vi "Set SPAN Component Lin.vi"(10 "LIN":T1, 11 "Lin Offset Cluster":T3) -> ()   [LabVIEW 2020, in "Linearisierung v2.lvlib" / "SpanEinstellungen.lvlib"]
uses:
  SpanEinstellungen.lvlib
  Auswahl Polynom Ordnung.ctl
  Linearisierung v2.lvlib
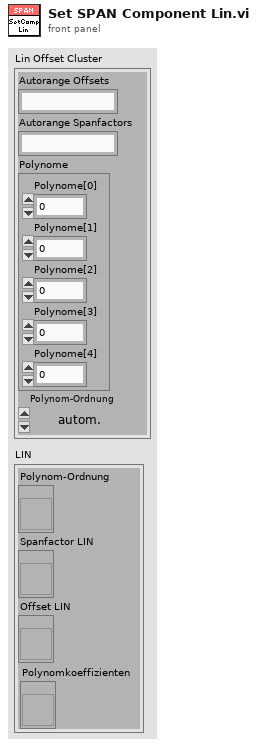
[diagram p1: front panel]
types:
  T1 = cluster{"Polynom-Ordnung":refnum<vi>, "Spanfactor LIN":refnum<vi>, "Offset LIN":refnum<vi>, "Polynomkoeffizienten":refnum<vi>}
  T2 = typedef "Linearisierung v2.lvlib/Auswahl Polynom Ordnung.ctl" = enum16{"autom.", "raw", "actual", "1", "2", "3", "4"}
  T3 = cluster{"Autorange Offsets":string, "Autorange Spanfactors":string, "Polynome":cluster{"Polynome[0]":dbl, "Polynome[1]":dbl, "Polynome[2]":dbl, "Polynome[3]":dbl, "Polynome[4]":dbl}, "Polynom-Ordnung":T2}
  T4 = cluster{"Polynome[0]":dbl, "Polynome[1]":dbl, "Polynome[2]":dbl, "Polynome[3]":dbl, "Polynome[4]":dbl}
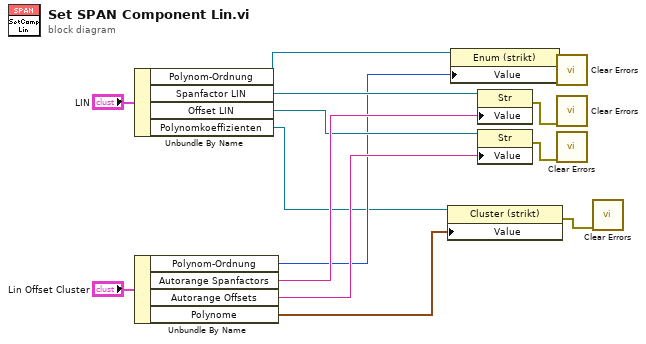
[diagram p0: block diagram]
diagram:
  n1 = Unbundle By Name("LIN") -> ("Polynom-Ordnung"=w6:refnum<vi>, "Spanfactor LIN"=w14:refnum<vi>, "Offset LIN"=w12:refnum<vi>, "Polynomkoeffizienten"=w3:refnum<vi>)
  n2 = Unbundle By Name("Lin Offset Cluster") -> ("Polynom-Ordnung"=w5:T2, "Autorange Spanfactors"=w13:string, "Autorange Offsets"=w11:string, "Polynome"=w1:T4)
  n3 = property class="Cluster (strikt)"(reference=w3, "Value"=w1) -> (error out=w2:errorcluster)  [unwired: 1 in, 1 out]
  n4 = property class="Enum (strikt)"(reference=w6, "Value"=w5) -> (error out=w7:errorcluster)  [unwired: 1 in, 1 out]
  n5 = property class="Str"(reference=w14, "Value"=w13) -> (error out=w10:errorcluster)  [unwired: 1 in, 1 out]
  n6 = property class="Str"(reference=w12, "Value"=w11) -> (error out=w9:errorcluster)  [unwired: 1 in, 1 out]
  n7 = call <vilib>:"Clear Errors.vi"("error in (no error)"=w7) -> ()  [unwired: 5 in, 2 out]
  n8 = call <vilib>:"Clear Errors.vi"("error in (no error)"=w10) -> ()  [unwired: 5 in, 2 out]
  n9 = call <vilib>:"Clear Errors.vi"("error in (no error)"=w9) -> ()  [unwired: 5 in, 2 out]
  n10 = call <vilib>:"Clear Errors.vi"("error in (no error)"=w2) -> ()  [unwired: 5 in, 2 out]
